vi "Parse Mobile Name.vi"(8 "error in (no error)":errorcluster, 11 "SSID in":string="Justin’s iPhone") -> (0 "error out":errorcluster, 2 "Justin's Phone":bool=TRUE, 3 "SSID out":string="Justin's iPhone")   [LabVIEW 2024]
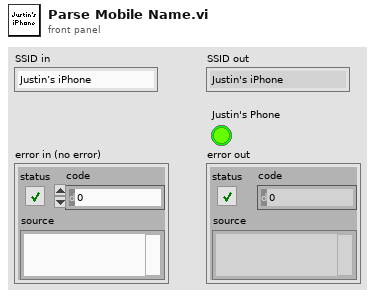
[diagram p1: front panel]
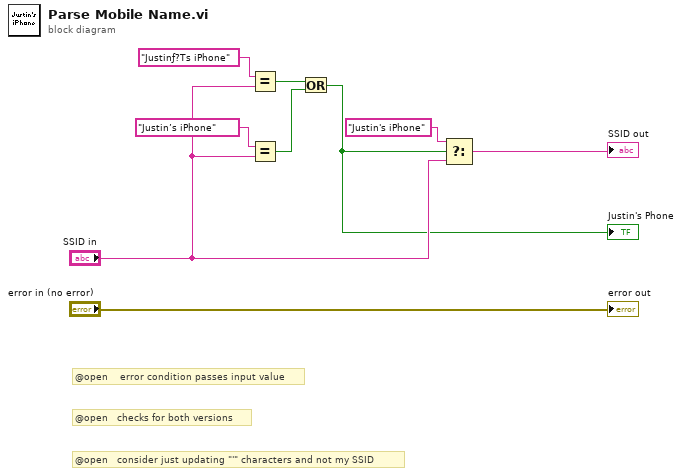
[diagram p0: block diagram]
diagram:
  # "@open   consider just updating \"'\" characters and not my SSID"
  # "@open   checks for both versions"
  # "@open    error condition passes input value"
  n1 = Equal?(x="Justinƒ?Ts iPhone" ("y"), y="SSID in") -> (x = y?=w3:bool)
  n2 = Equal?(x="Justin’s iPhone" ("y"), y="SSID in") -> (x = y?=w2:bool)
  n3 = Or(x=w3, y=w2) -> (x .or. y?=w1:bool)
  "Justin's Phone" <- w1
  n4 = Select(t="Justin's iPhone" ("y"), s=w1, f="SSID in") -> (s? t:f=→"SSID out":string)
  "error out" <- "error in (no error)"
